vi "CSV - Add New Columns.vi"(8 "error in (no error)":errorcluster, 9 "LV Data Types":T1[](array[typedef]) format="%.0x", 10 "Headers":string[](array[string]), 11 "TableLogger_CSV_Actor in":refnum<class "TableLogger_CSV_Actor.lvclass">) -> (0 "error out":errorcluster, 3 "TableLogger_CSV_Actor out":refnum<class "TableLogger_CSV_Actor.lvclass">)   [LabVIEW 2014, in "TableLogger_CSV_Actor.lvlib" / "TableLogger_CSV_Actor.lvclass"]
uses:
  TableLogger_CSV_Actor.lvclass
  <userlib>/_OpenG.lib/lvdata/lvdata.llb/Type Descriptor Enumeration__ogtk.ctl
  TableLogger_CSV_Actor.lvclass/TableLogger_CSV_Actor.ctl
panel:
  # "Connector Pane"
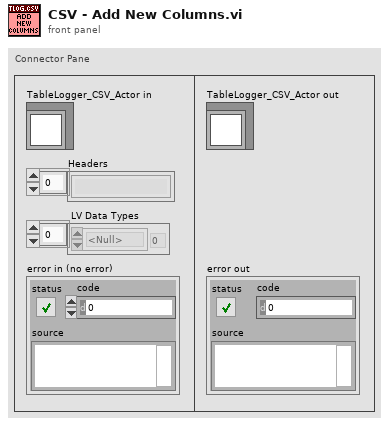
[diagram p1: front panel]
types:
  T1 = typedef "Type Descriptor Enumeration__ogtk.ctl" = enum8{"<Null>", "I8", "I16", "I32", "I64", "U8", "U16", "U32", "U64", "SGL", "DBL", "EXT", "CSG", "CDB", "CXT", "0x0F", "0x10", "0x11", "0x12", "0x13", "0x14", "Enum U8", "Enum U16", "Enum U32", "Enum U64", "SGL PQ", "DBL PQ", "EXT PQ", "CSG PQ", "CDB PQ", "CXT PQ", "0x1F", "0x20", "Boolean", "0x22", "0x23", "0x24", "0x25", "0x26", "0x27", "0x28", "0x29", "0x2A", "0x2B", "0x2C", "0x2D", "0x2E", "0x2F", "String", "0x31", "Path", "Pict", "0x34", "0x35", "0x36", "DAQ", "0x38", "0x39", "0x3A", "0x3B", "0x3C", "0x3D", "0x3E", "0x3F", "Array", "0x41", "0x42", "0x43", "0x44", "0x45", "0x46", "0x47", "0x48", "0x49", "0x4A", "0x4B", "0x4C", "0x4D", "0x4E", "0x4F", "Cluster", "0x51", "0x52", "Variant", "Waveform", "0x55", "0x56", "0x57", "0x58", "0x59", "0x5A", "0x5B", "0x5C", "0x5D", "0x5E", "0x5F", "0x60", "0x61", "0x62", "0x63", "0x64", "0x65", "0x66", "0x67", "0x68", "0x69", "0x6A", "0x6B", "0x6C", "0x6D", "0x6E", "0x6F", "Refnum"}
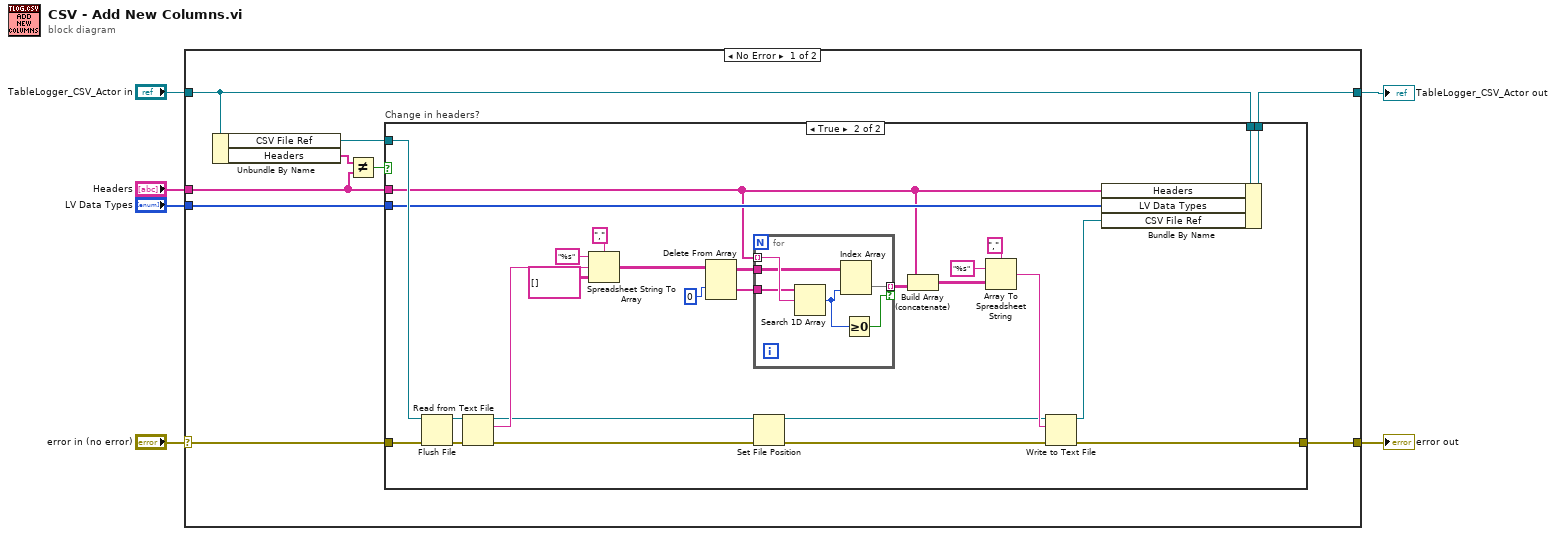
[diagram p0: block diagram]
diagram:
  n1 = case shown="No Error" "error in (no error)" {
    selector: "error in (no error)" -> [w13 w51]
    tunnel: [w15 w52] -> w6
    tunnel: "Headers" -> [w8 _]
    tunnel: "LV Data Types" -> [w10 _]
    tunnel: [w11 w51] -> w2
    tunnel: "TableLogger_CSV_Actor in" -> [w14 w52]
    frame No Error {
      n2 = Unbundle By Name(w14) -> ("CSV File Ref"=w12:refnum<file>, "Headers"=w9:string[])
      n3 = Not Equal?(x=w9, y=w8) -> (x != y?=w7:bool)
      n4 = case "Change in headers?" shown="True" w7 {
        tunnel: [w17 w44] -> w15
        tunnel: w14 -> [w17 w43]
        tunnel: w13 -> [w16 w42]
        tunnel: w12 -> [_ w39]
        tunnel: [w16 w29] -> w11
        tunnel: w10 -> [_ w23]
        tunnel: w8 -> [_ w21]
        frame False {
        }
        frame True {
          n5 = Flush File(refnum=w39, error in=w42) -> (refnum out=w38:refnum<file>, error out=w40:errorcluster)
          n6 = Read from Text File(file (use dialog)=w38, error in=w40) -> (refnum out=w19:refnum<file>, text=w37:string, error out=w41:errorcluster)  [unwired: 2 in, 1 out]
          n7 = Spreadsheet String To Array(delimiter (Tab)=",", format string="%s", spreadsheet string=w37, array type (2D Dbl)=string[][] []) -> (array=w33:string[][])
          n8 = Delete From Array(array=w33, index (row)=0) -> (deleted portion=w30:string[], array with subset deleted=w31:string[][])  [unwired: 2 in]
          n9 = for {
            tunnel: w31 -> [w48]
            tunnel: w30 -> [w49]
            tunnel: w21 -> [w50] mode=indexing
            tunnel: [w47] -> w26 mode=indexing if=w46
            n10 = Search 1D Array(1D array=w49, element=w50) -> (index of element=w45:i32)  [unwired: 1 in]
            n11 = Index Array(array=w48, index (col)=w45) -> (element=w47:string[])  [unwired: 1 in]
            n12 = Greater Or Equal To 0?(x=w45) -> (x >= 0?=w46:bool)
          }
          n13 = Set File Position(refnum=w19, error in=w41) -> (refnum out=w18:refnum<file>, error out=w20:errorcluster)  [unwired: 2 in]
          n14 = Build Array (concatenate)(w21, w26) -> (w22:string[][])
          n15 = Array To Spreadsheet String(delimiter (Tab)=",", array=w22, 3:"%s" ("format string")) -> (spreadsheet string=w27:string)
          n16 = Write to Text File(file (use dialog)=w18, text=w27, error in=w20) -> (refnum out=w28:refnum<file>, error out=w29:errorcluster)  [unwired: 1 in, 1 out]
          n17 = Bundle By Name(cluster=w43, "Headers"=w21, "LV Data Types"=w23, "CSV File Ref"=w28) -> (w44:refnum<class "TableLogger_CSV_Actor.lvclass">)
        }
      }
    }
    frame Error {
    }
  }
  "TableLogger_CSV_Actor out" <- w6
  "error out" <- w2
